vi "Create DFS Maze.vi"(10 "Height":i32, 11 "Width":i32) -> (3 "Maze":refnum<class "Maze.lvclass">)   [LabVIEW 2020, in "Maze.lvlib" / "MazeGen.lvclass"]
uses:
  MazeGen.lvclass
  Maze/Maze.lvclass
  Adjacency.ctl
  Position.ctl
  Maze.lvlib
panel:
  in  "Delay":u32=300
  in  "Preview":bool
  out "Preview":T1[][](array[typedef])
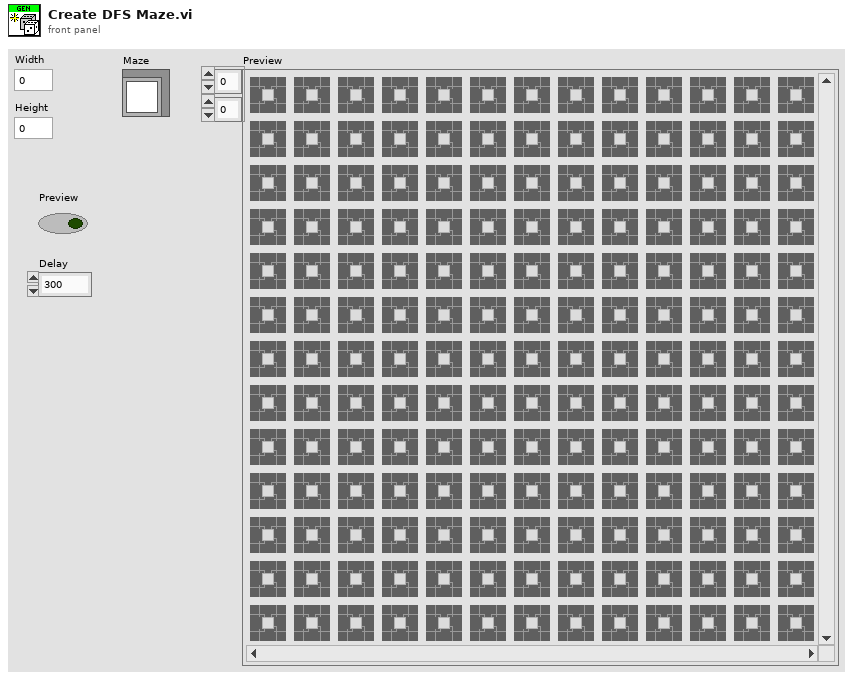
[diagram p1: front panel]
types:
  T1 = typedef "Maze.lvlib/Adjacency.ctl" = cluster{"E":bool, "N":bool, "W":bool, "S":bool, "Goal":bool, "Start":bool}
  T2 = typedef "Maze.lvlib/Position.ctl" = cluster{"S":i32, "E":i32}
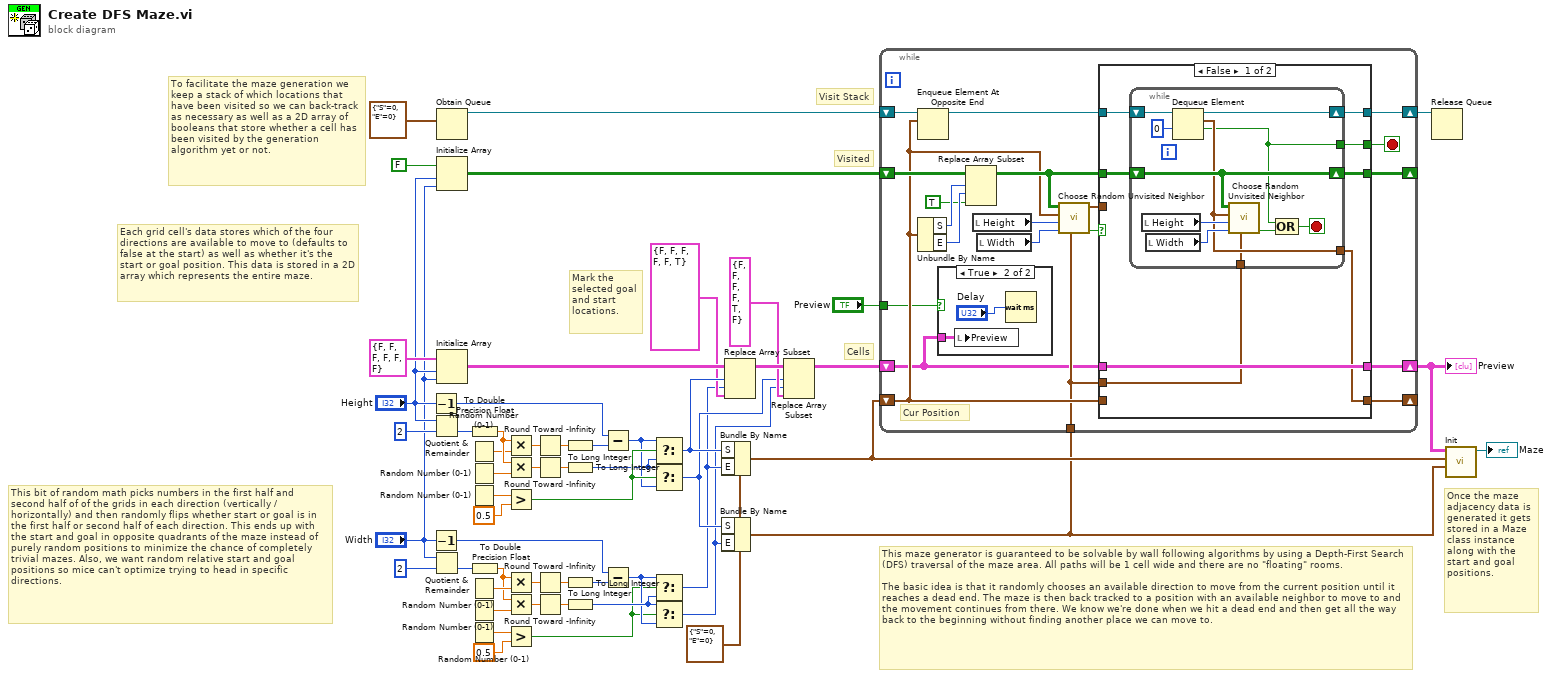
[diagram p0: block diagram]
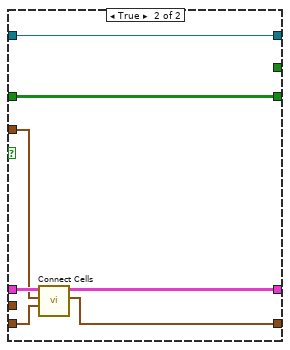
[diagram p3: hidden frame]
diagram:
  w27 = T2 {"S"=0, "E"=0} ("Position")
  # "Once the maze adjacency data is generated it gets stored in a Maze class instance along with the start and goal positions."
  # "Mark the selected goal and start locations."
  # "To facilitate the maze generation we keep a stack of which locations that have been visited so we can back-track as necessary as well as a 2D array of booleans that store whether a cell has been visited by the generation algorithm yet or not."
  # "Each grid cell's data stores which of the four directions are available to move to (defaults to false at the start) as well as whether it's the start or goal position. This data is stored in a 2D array which represents the entire maze."
  # "This maze generator is guaranteed to be solvable by wall following algorithms by using a Depth-First Search (DFS) traversal of the maze area. All paths will be 1 cell wide and there are no \"floating\" rooms.\n\nThe basic idea is that it randomly chooses an available direction to move from the current position until it reaches a dead end. The maze is then back tracked to a position with an available neighbor to move to and the movement continues from there. We know we're done when we hit a dead end and then get all the way back to the beginning without finding another place we can move to."
  # "This bit of random math picks numbers in the first half and second half of of the grids in each direction (vertically / horizontally) and then randomly flips whether start or goal is in the first half or second half of each direction. This ends up with the start and goal in opposite quadrants of the maze instead of purely random positions to minimize the chance of completely trivial mazes. Also, we want random relative start and goal positions so mice can't optimize trying to head in specific directions."
  # "Visit Stack"
  # "Visited"
  # "Cells"
  n1 = Decrement(x="Height") -> (x-1=w35:i32)
  n2 = Decrement(x="Width") -> (x-1=w45:i32)
  n3 = Quotient & Remainder(x="Height", y=2) -> (floor(x/y)=w30:i32)  [unwired: 1 out]
  n4 = Quotient & Remainder(x="Width", y=2) -> (floor(x/y)=w53:i32)  [unwired: 1 out]
  n5 = Obtain Queue(element data type=T2 {"S"=0, "E"=0} ("Position")) -> (queue out=w17:refnum<queue>)  [unwired: 4 in, 2 out]
  n6 = Initialize Array(FALSE, "Height", "Width") -> (w16:bool[][])
  n7 = Initialize Array(T1 {"E"=FALSE, "N"=FALSE, "W"=FALSE, "S"=FALSE, "Goal"=FALSE, "Start"=FALSE} ("Adjacency"), "Height", "Width") -> (w11:T1[][])
  n8 = Random Number (0-1)() -> (number: 0 to 1=w31:dbl)
  n9 = Random Number (0-1)() -> (number: 0 to 1=w32:dbl)
  n10 = Random Number (0-1)() -> (number: 0 to 1=w36:dbl)
  n11 = Random Number (0-1)() -> (number: 0 to 1=w52:dbl)
  n12 = Random Number (0-1)() -> (number: 0 to 1=w51:dbl)
  n13 = Random Number (0-1)() -> (number: 0 to 1=w44:dbl)
  n14 = To Double Precision Float(number=w30) -> (double precision float=w33:dbl)
  n15 = To Double Precision Float(number=w53) -> (double precision float=w50:dbl)
  n16 = Multiply(x=w33, y=w31) -> (x*y=w23:dbl)
  n17 = Multiply(x=w33, y=w32) -> (x*y=w22:dbl)
  n18 = Greater?(x=w36, y=0.5) -> (0:w39:bool)
  n19 = Multiply(x=w50, y=w52) -> (x*y=w25:dbl)
  n20 = Multiply(x=w50, y=w51) -> (x*y=w47:dbl)
  n21 = Greater?(x=w44, y=0.5) -> (0:w40:bool)
  n22 = Round Toward -Infinity(1:w23) -> (0:w20:dbl)
  n23 = Round Toward -Infinity(1:w22) -> (0:w21:dbl)
  n24 = Round Toward -Infinity(1:w25) -> (0:w24:dbl)
  n25 = Round Toward -Infinity(1:w47) -> (0:w26:dbl)
  n26 = To Long Integer(number=w20) -> (32bit integer=w34:i32)
  n27 = To Long Integer(number=w21) -> (32bit integer=w37:i32)
  n28 = To Long Integer(number=w24) -> (32bit integer=w46:i32)
  n29 = To Long Integer(number=w26) -> (32bit integer=w42:i32)
  n30 = Subtract(x=w35, y=w34) -> (x-y=w38:i32)
  n31 = Subtract(x=w45, y=w46) -> (x-y=w41:i32)
  n32 = Select(t=w38, s=w39, f=w37) -> (s? t:f=w10:i32)
  n33 = Select(t=w37, s=w39, f=w38) -> (s? t:f=w6:i32)
  n34 = Select(t=w41, s=w40, f=w42) -> (s? t:f=w5:i32)
  n35 = Select(t=w42, s=w40, f=w41) -> (s? t:f=w3:i32)
  n36 = Bundle By Name(cluster=w27, "S"=w10, "E"=w5) -> (w13:T2)
  n37 = Bundle By Name(cluster=w27, "S"=w6, "E"=w3) -> (w2:T2)
  n38 = Replace Array Subset(array=w11, new element=T1 {"E"=FALSE, "N"=FALSE, "W"=FALSE, "S"=FALSE, "Goal"=FALSE, "Start"=TRUE} ("new element/subarray"), index (row)=w10, index (col)=w5) -> (w8:T1[][])
  n39 = Replace Array Subset(array=w8, new element=T1 {"E"=FALSE, "N"=FALSE, "W"=FALSE, "S"=FALSE, "Goal"=TRUE, "Start"=FALSE} ("new element/subarray"), index (row)=w6, index (col)=w3) -> (w4:T1[][])
  n40 = while {
    shift-right: [w64] -> _
    shift-left: w13 -> [w60]
    shift-right: [w61] -> w15
    shift-left: w17 -> [w71]
    shift-right: [w62] -> _
    shift-left: w16 -> [w75]
    shift-right: [w63] -> w14
    shift-left: w4 -> [w57]
    tunnel: w2 -> [w58]
    tunnel: "Preview" -> [w56]
    stop <- w59 stop-if-true
    # "Cur Position"
    n41 = Enqueue Element At Opposite End(queue=w71, element=w60) -> (queue out=w66:refnum<queue>)  [unwired: 2 in, 2 out]
    n42 = Unbundle By Name(w60) -> ("S"=w74:i32, "E"=w73:i32)
    n43 = case shown="True" w56 {
      tunnel: w57 -> [_ w77]
      frame False {
      }
      frame True {
        n44 = local write "Preview"(w77) -> ()
        n45 = Wait (ms)(milliseconds to wait="Delay") -> ()  [unwired: 1 out]
      }
    }
    n46 = Replace Array Subset(array=w75, new element=TRUE ("new element/subarray"), index (row)=w74, index (col)=w73) -> (w65:bool[][])
    n47 = local read "Height"() -> (w70:i32)
    n48 = local read "Width"() -> (w69:i32)
    n49 = call "Choose Random Unvisited Neighbor.vi"("Goal"=w58, "Width"=w69, "Height"=w70, "Position"=w60, "Visited"=w65) -> ("Valid?"=w68:bool, "Random Unvisited Neighbor"=w67:T2)  [unwired: 5 in]
    n50 = case shown="False" w68 {
      tunnel: w67 -> [_ w100]
      tunnel: w66 -> [w85 w97]
      tunnel: w65 -> [w84 w98]
      tunnel: w57 -> [w80 w102]
      tunnel: w60 -> [_ w101]
      tunnel: [w79 w100] -> w64
      tunnel: [w80 w99] -> w63
      tunnel: [w81 w98] -> w62
      tunnel: [w82 w97] -> w61
      tunnel: [w83 _] -> w59
      tunnel: w58 -> [w78 _]
      frame False {
        n51 = while {
          shift-right: [w94] -> w82
          shift-left: w85 -> [w96]
          shift-right: [w93] -> w81
          shift-left: w84 -> [w93]
          tunnel: [w89] -> w83
          tunnel: [w90] -> w79
          tunnel: w78 -> [w86]
          stop <- w87 stop-if-true
          n52 = local read "Height"() -> (w92:i32)
          n53 = local read "Width"() -> (w91:i32)
          n54 = Dequeue Element(queue=w96, timeout in ms (-1)=0) -> (queue out=w94:refnum<queue>, element=w90:T2, timed out?=w89:bool)  [unwired: 1 in, 1 out]
          n55 = call "Choose Random Unvisited Neighbor.vi"("Goal"=w86, "Width"=w91, "Height"=w92, "Position"=w90, "Visited"=w93) -> ("Valid?"=w88:bool)  [unwired: 5 in, 1 out]
          n56 = Compound Arithmetic op=OR(w89, w88) -> (w87:bool)
        }
      }
      frame True {
        n57 = call "Connect Cells.vi"("To"=w101, "From"=w100, "Adjacency In"=w102) -> ("Adjacency"=w99:T1[][])  [unwired: 8 in]
      }
    }
  }
  "Preview" <- w14
  n58 = Release Queue(queue=w15) -> ()  [unwired: 2 in, 3 out]
  n59 = call "Init.vi"("Goal"=w2, "Start"=w13, "Adjacency"=w14) -> ("Maze out"=→"Maze":refnum<class "Maze.lvclass">)  [unwired: 7 in, 1 out]
